vi "Kikusui PLZ-Query Operation.vi"(8 "error in":errorcluster, 11 "Kikusui PLZ Setting In":T1={"VISA Resource Name"="", "Baud Rate"=19200, "Stop Bits"=20, "Wait For Read(ms)"=0} {"Stop Bits" items=["1.0"=10, "2.0"=20]; "Baud Rate" items=["2400"=2400, "4800"=4800, "9600"=9600, "19200"=19200]}) -> (0 "error out":errorcluster, 2 "Operation Mode":u16(ring) items=["Constant Current(CC)", "Constant Voltage(CV)", "Constant Power(CP)", "Constant Resistance(CR)", "Constant Current & Voltage(CCCV)", "Constant Resistance & Voltage(CRCV)"], 3 "Kikusui PLZ Setting Out":T1={"VISA Resource Name"="", "Baud Rate"=19200, "Stop Bits"=20, "Wait For Read(ms)"=0} {"Stop Bits" items=["1.0"=10, "2.0"=20]; "Baud Rate" items=["2400"=2400, "4800"=4800, "9600"=9600, "19200"=19200]})   [LabVIEW 2018]
uses:
  Data Def/Kikusui PLZ-Setting.ctl
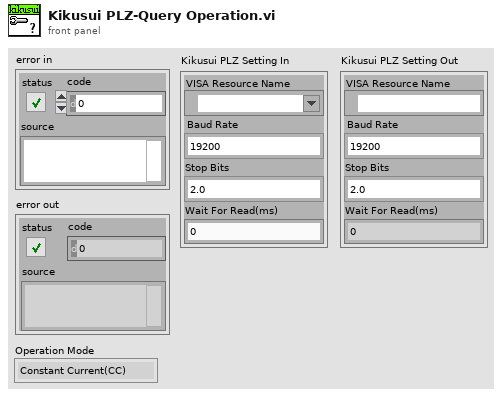
[diagram p1: front panel]
types:
  T1 = typedef "Kikusui PLZ-Setting.ctl" = cluster{"VISA Resource Name":refnum<visa-resource-name>, "Baud Rate":u32, "Stop Bits":u16, "Wait For Read(ms)":u32}
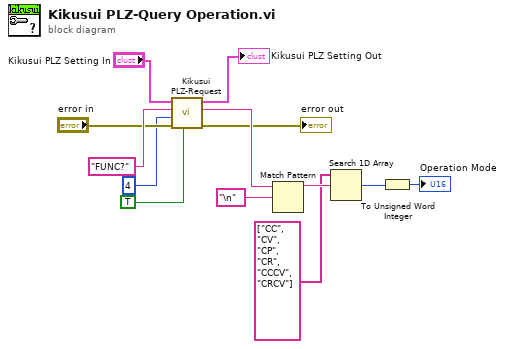
[diagram p0: block diagram]
diagram:
  n1 = call "Kikusui PLZ-Request.vi"("Response?"=TRUE, "error in"="error in", "byte count"=u32 4, "Command"="FUNC?", "Kikusui PLZ Setting In"="Kikusui PLZ Setting In") -> ("error out"=→"error out":errorcluster, "Response"=w9:string, "Kikusui PLZ Setting Out"=→"Kikusui PLZ Setting Out":T1)  [unwired: 4 in]
  n2 = Match Pattern(string=w9, regular expression="\n") -> (before substring=w7:string)  [unwired: 1 in, 3 out]
  n3 = Search 1D Array(1D array=string[] ["CC", "CV", "CP", "CR", "CCCV", "CRCV"], element=w7) -> (index of element=w5:i32)  [unwired: 1 in]
  n4 = To Unsigned Word Integer(number=w5) -> (unsigned 16bit integer=→"Operation Mode":u16)
